vi "Set Error.vi"(9 "Is Override":bool, 10 "Error":errorcluster, 11 "Base Actor in":refnum<class "Base Actor.lvclass">) -> (3 "Base Actor out":refnum<class "Base Actor.lvclass">)   [LabVIEW 2020, in "jettl.lvlib" / "Actor.lvlib" / "Base Actor.lvclass"]
uses:
  Base Actor.lvclass
  Base Actor.lvclass/Base Actor.ctl
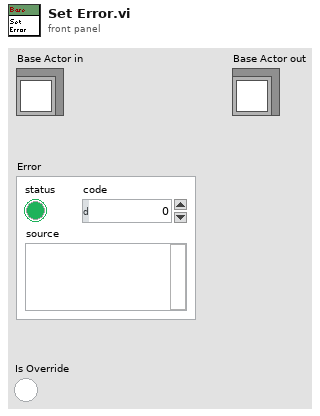
[diagram p1: front panel]
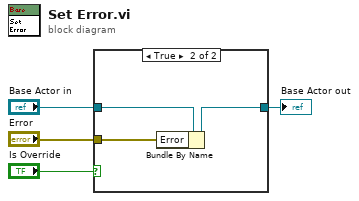
[diagram p0: block diagram]
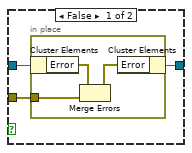
[diagram p2: hidden frame]
diagram:
  n1 = case shown="True" "Is Override" {
    tunnel: "Base Actor in" -> [w7 w12]
    tunnel: [w6 w11] -> w2
    tunnel: "Error" -> [w5 w13]
    frame False {
      n2 = in-place {
        in-place-border: w5 -> [w9]
        n3 = in-place-cluster #1(w7) -> ("Error"=w10:errorcluster)
        n4 = Merge Errors(w10, w9) -> (w8:errorcluster)
        n5 = in-place-cluster #1("Error"=w8) -> (w6:refnum<class "Base Actor.lvclass">)
      }
    }
    frame True {
      n6 = Bundle By Name(cluster=w12, "Error"=w13) -> (w11:refnum<class "Base Actor.lvclass">)
    }
  }
  "Base Actor out" <- w2
